vi "Engine-AnalogInput.vi"(8 "error in (no error)":errorcluster, 11 "DSI Reference":refnum<class "DCM-DSI.lvclass">) -> (0 "error out":errorcluster, 3 "DSI Reference":refnum<class "DCM-DSI.lvclass">)   [LabVIEW 2016, in "DSI-RT.lvlib"]
uses:
  DSI-RT.lvlib
  Classes/DCM-DSI/DCM-DSI.lvclass
  <vilib>/addons/Software Calibration Management/xSCM/Controls/TBL1D.ctl
  Classes/DCM-DSI/Read System ADC.vi
  Classes/DCM-DSI/Read dt.vi
  Classes/DCM-DSI/Write Channels.vi
  <vilib>/addons/Software Calibration Management/xSCM/CalPoint.xnode
  <vilib>/addons/Software Calibration Management/xSCM/SCM-API.lvlib
  <vilib>/addons/Software Calibration Management/xSCM/ni_scm.dll
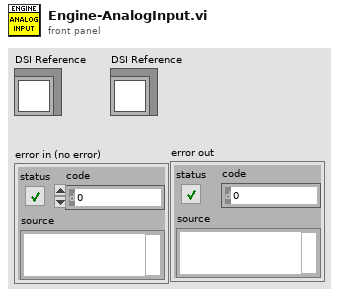
[diagram p1: front panel]
types:
  T1 = typedef "DCM - RT.lvclass/System ADC.ctl" = cluster{"AI 1 [V]":sgl, "AI 2 [V]":sgl, "AI 3 [V]":sgl, "AI 4 [V]":sgl, "AI 5 [V]":sgl, "AI 6 [V]":sgl, "AI 7 [V]":sgl, "AI 8 [V]":sgl, "AI 9 [V]":sgl, "AI 10 [V]":sgl, "AI 11 [V]":sgl, "AI 12 [V]":sgl, "Temp HH 1-6 [C]":sgl, "Temp HH 7-12 [C]":sgl, "Temp DI A [C]":sgl, "Temp DI Zener A [C]":sgl, "Temp DI B [C]":sgl, "Temp DI Zener B [C]":sgl, "Temp CPU [C]":sgl, "Temp Fan Intake [C]":sgl, "Temp Secondary A [C]":sgl, "Temp Primary A [C]":sgl, "Temp Boost B [C]":sgl, "Primary Range [V]":sgl, "Primary A1A2 [V]":sgl, "Primary A3A4 [V]":sgl, "Primary B3B4 [V]":sgl, "Primary B1B2 [V]":sgl, "Secondary A1A2 [V]":sgl, "Secondary A3A4 [V]":sgl, "Secondary B3B4 [V]":sgl, "Secondary B1B2 [V]":sgl, "Ext HV A [V]":sgl, "Ext HV B [V]":sgl, "FET Driver [V]":sgl, "Fan [V]":sgl, "Battery [V]":sgl, "DRVP [V]":sgl, "Key [V]":sgl, "DI Zener A [V]":sgl, "DI Zener B [V]":sgl, "Pump Zener A [V]":sgl, "Pump Zener B [V]":sgl, "MPRD [V]":sgl}
  T2 = typedef "SCM-API.lvlib/TBL1D.ctl" = cluster{"X":sgl[], "Y":sgl[]}
  T3 = cluster{"String":string, "String":string, "Numeric":sgl, bool, bool, "Numeric":sgl, "Numeric":sgl, "Value":T2}
  T4 = typedef "DSI-Shared.lvlib/Engine-Channel.ctl" = cluster{"Name":string, "Unit":string, "Value":sgl}
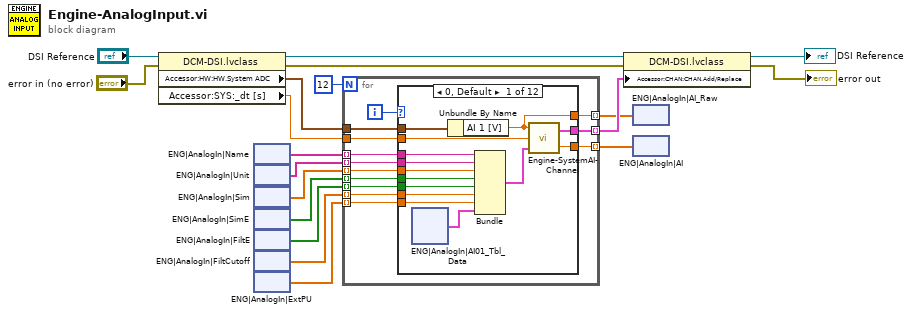
[diagram p0: block diagram]
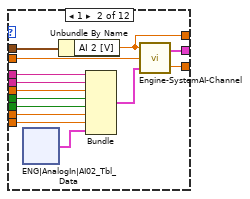
[diagram p2: hidden frame]
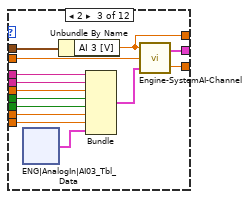
[diagram p3: hidden frame]
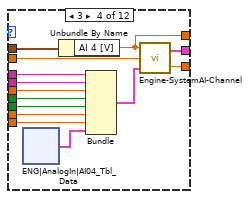
[diagram p4: hidden frame]
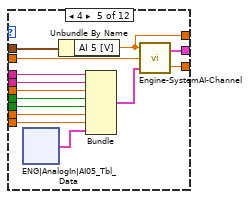
[diagram p5: hidden frame]
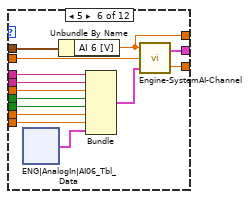
[diagram p6: hidden frame]
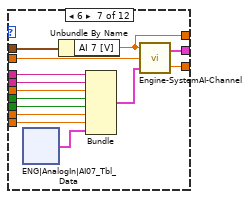
[diagram p7: hidden frame]
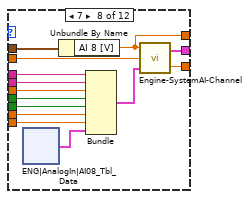
[diagram p8: hidden frame]
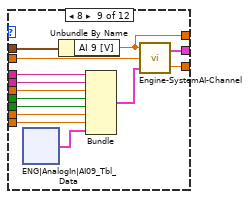
[diagram p9: hidden frame]
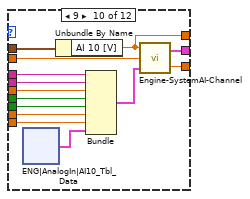
[diagram p10: hidden frame]
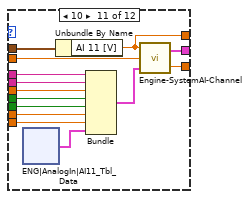
[diagram p11: hidden frame]
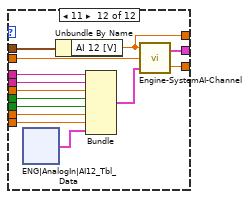
[diagram p12: hidden frame]
diagram:
  n1 = property class="DCM-DSI.lvclass"(reference="DSI Reference", error in="error in (no error)") -> (reference out=w17:refnum<class "DCM-DSI.lvclass">, error out=w12:errorcluster, "Accessor:HW:HW.System ADC"=w11:T1, "Accessor:SYS:_dt [s]"=w14:sgl)
  n2 = xnode "ENG|AnalogIn|Name"() -> ("Value"=w9:string[])
  n3 = xnode "ENG|AnalogIn|Unit"() -> ("Value"=w8:string[])
  n4 = xnode "ENG|AnalogIn|Sim"() -> ("Value"=w7:sgl[])
  n5 = xnode "ENG|AnalogIn|SimE"() -> ("Value"=w6:bool[])
  n6 = xnode "ENG|AnalogIn|FiltE"() -> ("Value"=w5:bool[])
  n7 = xnode "ENG|AnalogIn|FiltCutoff"() -> ("Value"=w4:sgl[])
  n8 = xnode "ENG|AnalogIn|ExtPU"() -> ("Value"=w3:sgl[])
  n9 = for {
    N: 12 -> [_]
    tunnel: w11 -> [w30]
    tunnel: w14 -> [w32]
    tunnel: [w29] -> w10 mode=indexing
    tunnel: w9 -> [w28] mode=indexing
    tunnel: w8 -> [w27] mode=indexing
    tunnel: w7 -> [w26] mode=indexing
    tunnel: w6 -> [w25] mode=indexing
    tunnel: w5 -> [w24] mode=indexing
    tunnel: w4 -> [w23] mode=indexing
    tunnel: w3 -> [w22] mode=indexing
    tunnel: [w21] -> w2 mode=indexing
    tunnel: [w20] -> w1 mode=indexing
    i -> [w31]
    n10 = case shown="0, Default" w31 {
      tunnel: w32 -> [w46 w73 w100 w127 w154 w181 w208 w235 w262 w289 w316 w343]
      tunnel: w30 -> [w45 w72 w99 w126 w153 w180 w207 w234 w261 w288 w315 w342]
      tunnel: [w44 w71 w98 w125 w152 w179 w206 w233 w260 w287 w314 w341] -> w29
      tunnel: w28 -> [w42 w69 w96 w123 w150 w177 w204 w231 w258 w285 w312 w339]
      tunnel: w27 -> [w41 w68 w95 w122 w149 w176 w203 w230 w257 w284 w311 w338]
      tunnel: w26 -> [w40 w67 w94 w121 w148 w175 w202 w229 w256 w283 w310 w337]
      tunnel: w25 -> [w39 w66 w93 w120 w147 w174 w201 w228 w255 w282 w309 w336]
      tunnel: w24 -> [w38 w65 w92 w119 w146 w173 w200 w227 w254 w281 w308 w335]
      tunnel: w23 -> [w37 w64 w91 w118 w145 w172 w199 w226 w253 w280 w307 w334]
      tunnel: w22 -> [w36 w63 w90 w117 w144 w171 w198 w225 w252 w279 w306 w333]
      tunnel: [w33 w61 w88 w115 w142 w168 w196 w223 w250 w277 w304 w331] -> w21
      tunnel: [w34 w60 w87 w114 w141 w169 w195 w222 w249 w276 w303 w330] -> w20
      frame 0, Default {
        n11 = xnode "ENG|AnalogIn|AI01_Tbl_Data"() -> ("Value"=w35:T2)
        n12 = Unbundle By Name(w45) -> ("AI 1 [V]"=w33:sgl)
        n13 = Bundle("String"=w42, "String"=w41, "Numeric"=w40, w39, w38, "Numeric"=w37, "Numeric"=w36, "Value"=w35) -> (w43:T3)  [unwired: 1 in]
        n14 = call "Engine-SystemAI-Channel.vi"("Settings"=w43, "dt [s]"=w46, "AI [V]"=w33) -> (0:"AI"=w34:sgl, 1:"AI"=w44:T4)
      }
      frame 1 {
        n15 = xnode "ENG|AnalogIn|AI02_Tbl_Data"() -> ("Value"=w62:T2)
        n16 = Unbundle By Name(w72) -> ("AI 2 [V]"=w61:sgl)
        n17 = Bundle("String"=w69, "String"=w68, "Numeric"=w67, w66, w65, "Numeric"=w64, "Numeric"=w63, "Value"=w62) -> (w70:T3)  [unwired: 1 in]
        n18 = call "Engine-SystemAI-Channel.vi"("Settings"=w70, "dt [s]"=w73, "AI [V]"=w61) -> (0:"AI"=w60:sgl, 1:"AI"=w71:T4)
      }
      frame 2 {
        n19 = xnode "ENG|AnalogIn|AI03_Tbl_Data"() -> ("Value"=w89:T2)
        n20 = Unbundle By Name(w99) -> ("AI 3 [V]"=w88:sgl)
        n21 = Bundle("String"=w96, "String"=w95, "Numeric"=w94, w93, w92, "Numeric"=w91, "Numeric"=w90, "Value"=w89) -> (w97:T3)  [unwired: 1 in]
        n22 = call "Engine-SystemAI-Channel.vi"("Settings"=w97, "dt [s]"=w100, "AI [V]"=w88) -> (0:"AI"=w87:sgl, 1:"AI"=w98:T4)
      }
      frame 3 {
        n23 = xnode "ENG|AnalogIn|AI04_Tbl_Data"() -> ("Value"=w116:T2)
        n24 = Unbundle By Name(w126) -> ("AI 4 [V]"=w115:sgl)
        n25 = Bundle("String"=w123, "String"=w122, "Numeric"=w121, w120, w119, "Numeric"=w118, "Numeric"=w117, "Value"=w116) -> (w124:T3)  [unwired: 1 in]
        n26 = call "Engine-SystemAI-Channel.vi"("Settings"=w124, "dt [s]"=w127, "AI [V]"=w115) -> (0:"AI"=w114:sgl, 1:"AI"=w125:T4)
      }
      frame 4 {
        n27 = xnode "ENG|AnalogIn|AI05_Tbl_Data"() -> ("Value"=w143:T2)
        n28 = Unbundle By Name(w153) -> ("AI 5 [V]"=w142:sgl)
        n29 = Bundle("String"=w150, "String"=w149, "Numeric"=w148, w147, w146, "Numeric"=w145, "Numeric"=w144, "Value"=w143) -> (w151:T3)  [unwired: 1 in]
        n30 = call "Engine-SystemAI-Channel.vi"("Settings"=w151, "dt [s]"=w154, "AI [V]"=w142) -> (0:"AI"=w141:sgl, 1:"AI"=w152:T4)
      }
      frame 5 {
        n31 = xnode "ENG|AnalogIn|AI06_Tbl_Data"() -> ("Value"=w170:T2)
        n32 = Unbundle By Name(w180) -> ("AI 6 [V]"=w168:sgl)
        n33 = Bundle("String"=w177, "String"=w176, "Numeric"=w175, w174, w173, "Numeric"=w172, "Numeric"=w171, "Value"=w170) -> (w178:T3)  [unwired: 1 in]
        n34 = call "Engine-SystemAI-Channel.vi"("Settings"=w178, "dt [s]"=w181, "AI [V]"=w168) -> (0:"AI"=w169:sgl, 1:"AI"=w179:T4)
      }
      frame 6 {
        n35 = xnode "ENG|AnalogIn|AI07_Tbl_Data"() -> ("Value"=w197:T2)
        n36 = Unbundle By Name(w207) -> ("AI 7 [V]"=w196:sgl)
        n37 = Bundle("String"=w204, "String"=w203, "Numeric"=w202, w201, w200, "Numeric"=w199, "Numeric"=w198, "Value"=w197) -> (w205:T3)  [unwired: 1 in]
        n38 = call "Engine-SystemAI-Channel.vi"("Settings"=w205, "dt [s]"=w208, "AI [V]"=w196) -> (0:"AI"=w195:sgl, 1:"AI"=w206:T4)
      }
      frame 7 {
        n39 = xnode "ENG|AnalogIn|AI08_Tbl_Data"() -> ("Value"=w224:T2)
        n40 = Unbundle By Name(w234) -> ("AI 8 [V]"=w223:sgl)
        n41 = Bundle("String"=w231, "String"=w230, "Numeric"=w229, w228, w227, "Numeric"=w226, "Numeric"=w225, "Value"=w224) -> (w232:T3)  [unwired: 1 in]
        n42 = call "Engine-SystemAI-Channel.vi"("Settings"=w232, "dt [s]"=w235, "AI [V]"=w223) -> (0:"AI"=w222:sgl, 1:"AI"=w233:T4)
      }
      frame 8 {
        n43 = xnode "ENG|AnalogIn|AI09_Tbl_Data"() -> ("Value"=w251:T2)
        n44 = Unbundle By Name(w261) -> ("AI 9 [V]"=w250:sgl)
        n45 = Bundle("String"=w258, "String"=w257, "Numeric"=w256, w255, w254, "Numeric"=w253, "Numeric"=w252, "Value"=w251) -> (w259:T3)  [unwired: 1 in]
        n46 = call "Engine-SystemAI-Channel.vi"("Settings"=w259, "dt [s]"=w262, "AI [V]"=w250) -> (0:"AI"=w249:sgl, 1:"AI"=w260:T4)
      }
      frame 9 {
        n47 = xnode "ENG|AnalogIn|AI10_Tbl_Data"() -> ("Value"=w278:T2)
        n48 = Unbundle By Name(w288) -> ("AI 10 [V]"=w277:sgl)
        n49 = Bundle("String"=w285, "String"=w284, "Numeric"=w283, w282, w281, "Numeric"=w280, "Numeric"=w279, "Value"=w278) -> (w286:T3)  [unwired: 1 in]
        n50 = call "Engine-SystemAI-Channel.vi"("Settings"=w286, "dt [s]"=w289, "AI [V]"=w277) -> (0:"AI"=w276:sgl, 1:"AI"=w287:T4)
      }
      frame 10 {
        n51 = xnode "ENG|AnalogIn|AI11_Tbl_Data"() -> ("Value"=w305:T2)
        n52 = Unbundle By Name(w315) -> ("AI 11 [V]"=w304:sgl)
        n53 = Bundle("String"=w312, "String"=w311, "Numeric"=w310, w309, w308, "Numeric"=w307, "Numeric"=w306, "Value"=w305) -> (w313:T3)  [unwired: 1 in]
        n54 = call "Engine-SystemAI-Channel.vi"("Settings"=w313, "dt [s]"=w316, "AI [V]"=w304) -> (0:"AI"=w303:sgl, 1:"AI"=w314:T4)
      }
      frame 11 {
        n55 = xnode "ENG|AnalogIn|AI12_Tbl_Data"() -> ("Value"=w332:T2)
        n56 = Unbundle By Name(w342) -> ("AI 12 [V]"=w331:sgl)
        n57 = Bundle("String"=w339, "String"=w338, "Numeric"=w337, w336, w335, "Numeric"=w334, "Numeric"=w333, "Value"=w332) -> (w340:T3)  [unwired: 1 in]
        n58 = call "Engine-SystemAI-Channel.vi"("Settings"=w340, "dt [s]"=w343, "AI [V]"=w331) -> (0:"AI"=w330:sgl, 1:"AI"=w341:T4)
      }
    }
  }
  n59 = property class="DCM-DSI.lvclass"(reference=w17, error in=w12, "Accessor:CHAN:CHAN.Add/Replace"=w10) -> (reference out=→"DSI Reference":refnum<class "DCM-DSI.lvclass">, error out=→"error out":errorcluster)
  n60 = xnode "ENG|AnalogIn|AI_Raw"("Value"=w2) -> ()
  n61 = xnode "ENG|AnalogIn|AI"("Value"=w1) -> ()
